vi "ELVIS III v1.0 Config AI IRQ.vi"(3 "Hysteresis":dbl=0.02, 5 "Enable IRQ?":bool, 6 "Threshold":dbl=2.5, 7 "IRQ Number":u8, 8 "error in (no error)":errorcluster, 9 "IO IRQ Channels Enum":T1, 10 "IRQ Type":T3, 11 "myRIO FPGA Ref In":T2) -> (0 "error out":errorcluster)   [LabVIEW 2021]
uses:
  <vilib>/myRIO/Common/Instrument Driver Framework/myRIO v1.0/IRQ/typedefs/IRQ Type.ctl
  <vilib>/myRIO/Common/Instrument Driver Framework/Utilities/typedefs/Generic FPGA Reference.ctl
  <vilib>/myRIO/Common/Instrument Driver Framework/myRIO v1.0/IRQ/typedefs/IO IRQ Channels Enum.ctl
  <vilib>/myRIO/Common/Instrument Driver Framework/ELVIS III v1.0/IRQ/typedefs/ELVIS III AI IRQ Channels FPGA Reference.ctl
  <vilib>/Utility/error.llb/Error Cluster From Error Code.vi
  <vilib>/rvi/errors/niLvFpgaAdjustHostInterfaceError.vi
  <vilib>/rvi/interface/nirviReadWriteControl/nirviReadWriteControl.xnode
  <vilib>/rvi/interface/Simulation/niFpgaSimulationCallBeginRW.vi
  NiFpgaLv.dll
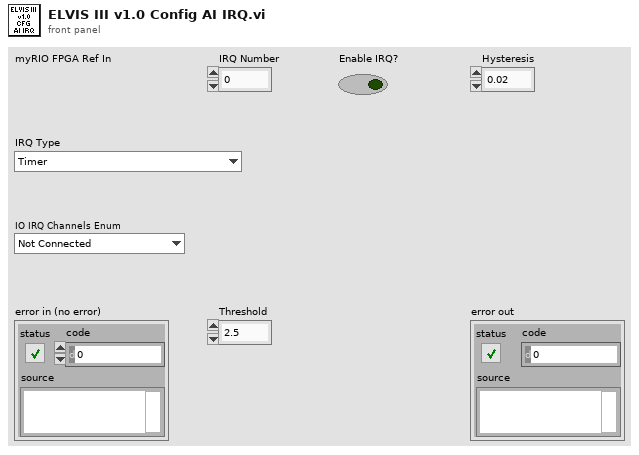
[diagram p1: front panel]
types:
  T1 = typedef "IO IRQ Channels Enum.ctl" = enum16{"Not Connected", "A/AI0 (Interrupt)", "A/AI1 (Interrupt)", "A/DIO0 (Interrupt)", "A/DIO1 (Interrupt)", "A/DIO2 (Interrupt)", "A/DIO3 (Interrupt)", "Button0 (Interrupt)", "B/AI0 (Interrupt)", "B/AI1 (Interrupt)", "B/DIO0 (Interrupt)", "B/DIO1 (Interrupt)", "B/DIO2 (Interrupt)", "B/DIO3 (Interrupt)"}
  T2 = typedef "Generic FPGA Reference.ctl" = refnum<k20>
  T3 = typedef "IRQ Type.ctl" = enum16{"Timer", "Analog falling edge", "Analog rising edge", "Digital falling edge", "Digital rising edge", "Digital edge"}
  T4 = typedef "ELVIS III AI IRQ Channels FPGA Reference.ctl" = refnum<k20>
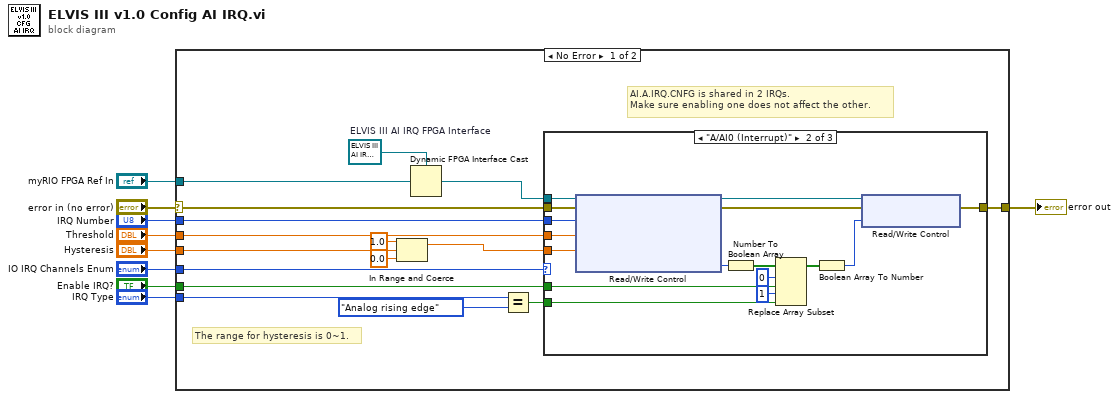
[diagram p0: block diagram]
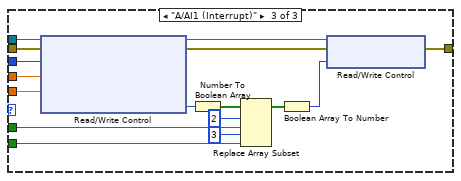
[diagram p3: hidden frame]
diagram:
  n1 = case shown="No Error" "error in (no error)" {
    selector: "error in (no error)" -> [w12 w59]
    tunnel: [w25 w59] -> w9
    tunnel: "IRQ Type" -> [w22 _]
    tunnel: "IRQ Number" -> [w18 _]
    tunnel: "myRIO FPGA Ref In" -> [w21 _]
    tunnel: "IO IRQ Channels Enum" -> [w16 _]
    tunnel: "Threshold" -> [w11 _]
    tunnel: "Enable IRQ?" -> [w17 _]
    tunnel: "Hysteresis" -> [w15 _]
    frame No Error {
      w19 = T4 refnum  # ELVIS III AI IRQ FPGA Interface
      # "AI.A.IRQ.CNFG is shared in 2 IRQs.\nMake sure enabling one does not affect the other."
      # "The range for hysteresis is 0~1."
      n2 = In Range and Coerce(upper limit=1.0, x=w15, lower limit=0.0) -> (coerced(x)=w10:dbl)  [unwired: 1 out]
      n3 = Dynamic FPGA Interface Cast(Session In=w19, Type=w21) -> (Session Out=w20:T4)
      n4 = Equal?(x=w22, y=IRQ_Type."Analog rising edge") -> (x = y?=w24:bool)
      n5 = case shown="\"A/AI0 (Interrupt)\"" w16 {
        tunnel: w24 -> [_ w31 w45]
        tunnel: w20 -> [_ w42 w57]
        tunnel: w18 -> [_ w41 w58]
        tunnel: w11 -> [_ w28 w44]
        tunnel: w12 -> [w26 w40 w56]
        tunnel: [w26 w37 w54] -> w25
        tunnel: w17 -> [_ w32 w46]
        tunnel: w10 -> [_ w27 w43]
        frame Default {
        }
        frame "A/AI0 (Interrupt)" {
          n6 = xnode "Read/Write Control"("FPGA VI Reference In"=w42, "error in"=w40, "IRQ.AI_A_0.NO"=w41, "IRQ.AI_A_0.THRESHOLD"=w28, "IRQ.AI_A_0.HYSTERESIS"=w27) -> ("FPGA VI Reference Out"=w38:T4, "error out"=w39:errorcluster, "IRQ.AI_A.CNFG"=w36:u8)
          n7 = Number To Boolean Array(number=w36) -> (Boolean array=w35:bool[])
          n8 = Replace Array Subset(array=w35, new element #1=w32, index #1=0 ("index"), new element #2=w31, index #2=1 ("index")) -> (w34:bool[])
          n9 = Boolean Array To Number(Boolean array=w34) -> (number=w33:u8)
          n10 = xnode "Read/Write Control"("FPGA VI Reference In"=w38, "error in"=w39, "IRQ.AI_A.CNFG"=w33) -> ("error out"=w37:errorcluster)  [unwired: 1 out]
        }
        frame "A/AI1 (Interrupt)" {
          n11 = xnode "Read/Write Control"("FPGA VI Reference In"=w57, "error in"=w56, "IRQ.AI_A_1.NO"=w58, "IRQ.AI_A_1.THRESHOLD"=w44, "IRQ.AI_A_1.HYSTERESIS"=w43) -> ("FPGA VI Reference Out"=w53:T4, "error out"=w55:errorcluster, "IRQ.AI_A.CNFG"=w50:u8)
          n12 = Number To Boolean Array(number=w50) -> (Boolean array=w52:bool[])
          n13 = Replace Array Subset(array=w52, new element #1=w46, index #1=2 ("index"), new element #2=w45, index #2=3 ("index")) -> (w51:bool[])
          n14 = Boolean Array To Number(Boolean array=w51) -> (number=w49:u8)
          n15 = xnode "Read/Write Control"("FPGA VI Reference In"=w53, "error in"=w55, "IRQ.AI_A.CNFG"=w49) -> ("error out"=w54:errorcluster)  [unwired: 1 out]
        }
      }
    }
    frame Error {
    }
  }
  "error out" <- w9
